vi "Read UTF-8 String.vi"(8 "error in (no error)":errorcluster, 11 "UTF8 in":refnum<class "UTF-8 String.lvclass">) -> (0 "error out":errorcluster, 2 "UTF-8 String":string, 3 "UTF8 out":refnum<class "UTF-8 String.lvclass">)   [LabVIEW 2019, in "JKI Unicode.lvlib" / "UTF-8 String.lvclass"]
doc: "JKI Unicode 1.0.0.7\nTomi Maila - JKI\nCopyright (c) 2016, JKI"
uses:
  UTF-8 String.lvclass
  UTF-8 String.lvclass/UTF-8 String.ctl
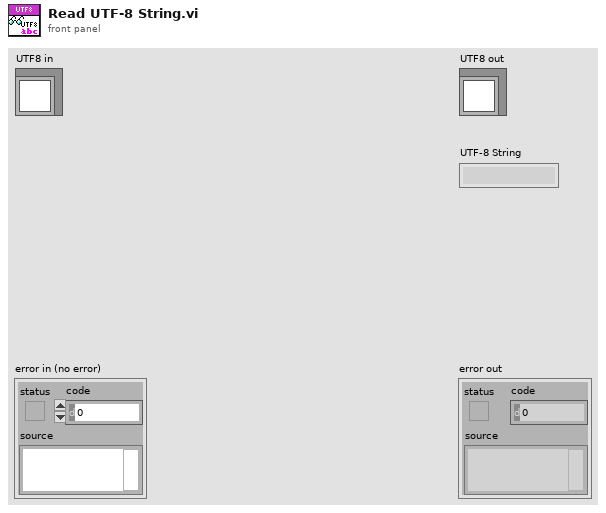
[diagram p1: front panel]
types:
  T1 = typedef "JKI Unicode.lvlib/UTF-8 String.lvclass/Byte Stream.ctl" = u8[]
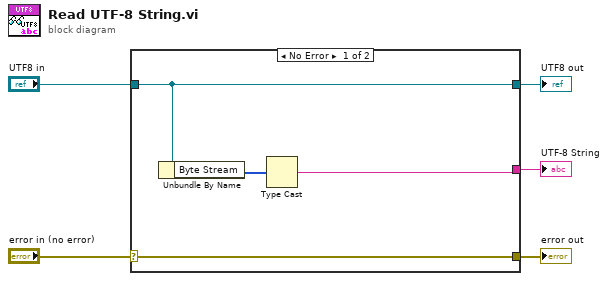
[diagram p0: block diagram]
diagram:
  n1 = case shown="No Error" "error in (no error)" {
    selector: "error in (no error)" -> [w9 w10]
    tunnel: [w9 w10] -> w4
    tunnel: [w8 w11] -> w2
    tunnel: "UTF8 in" -> [w8 w11]
    tunnel: [w6 _] -> w1
    frame No Error {
      n2 = Unbundle By Name(w8) -> ("Byte Stream"=w7:T1)
      n3 = Type Cast(x=w7) -> (*(type *) &x=w6:string)  [unwired: 1 in]
    }
    frame Error {
    }
  }
  "error out" <- w4
  "UTF8 out" <- w2
  "UTF-8 String" <- w1
